vi "BRig_RT_comm_webdav_upload_all__announceExpPrefix.vi"(6 "input_fileName_prefix":string, 10 "input_errro":errorcluster, 11 "intput_hSession":T1) -> (0 "output_checkData":bool, 2 "output_error":errorcluster, 3 "output_hSession":T1)   [LabVIEW 2014]
uses:
  <vilib>/WebDAVClient/Advanced/SessionHandle.ctl
  <vilib>/WebDAVClient/NI_WebDAV.lvlib
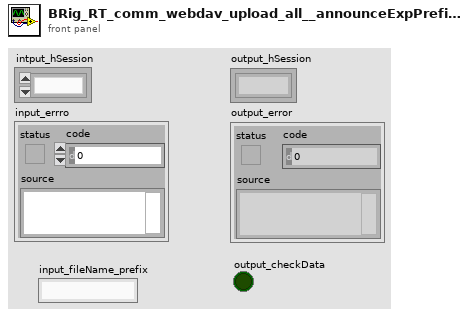
[diagram p1: front panel]
types:
  T1 = typedef "NI_WebDAV.lvlib/SessionHandle.ctl" = refnum<k1>
  T2 = enum16{"open", "replace", "create", "open or create", "replace or create", "replace or create with confirmation"}
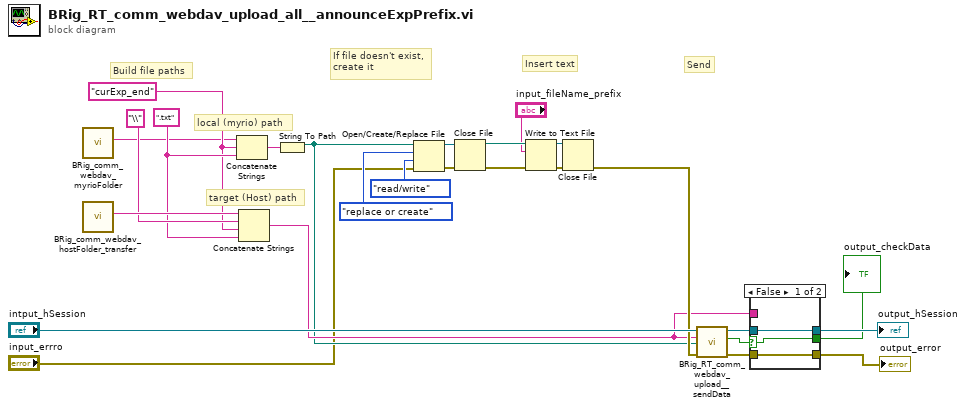
[diagram p0: block diagram]
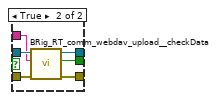
[diagram p2: hidden frame]
diagram:
  w22 = "curExp_end" ("intput_fileName")
  w23 = ".txt" ("string")
  # "Send"
  # "Insert text"
  # "If file doesn't exist,\ncreate it"
  # "local (myrio) path"
  # "target (Host) path"
  # "Build file paths"
  n1 = call "BRig_comm_webdav_myrioFolder.vi"() -> ("output_myrioFolder"=w21:string)  [unwired: 11 in]
  n2 = call "BRig_comm_webdav_hostFolder_transfer.vi"() -> ("output_HostFolder"=w25:string)  [unwired: 11 in]
  n3 = Concatenate Strings(w21, w22, w23) -> (w26:string)
  n4 = Concatenate Strings(w25, "\\" ("string"), w22, w23) -> (w10:string)
  n5 = String To Path(string=w26) -> (path=w2:path)
  n6 = Open/Create/Replace File(file path (use dialog)=w2, error in="input_errro", operation (0:open)=T2."replace or create", access (0:read/write)=enum16{"read/write", "read-only", "write-only"}."read/write") -> (refnum out=w3:refnum<file>, error out=w4:errorcluster)  [unwired: 2 in, 1 out]
  n7 = Close File(refnum=w3, error in=w4) -> (path=w17:path, error out=w18:errorcluster)
  n8 = Write to Text File(file (use dialog)=w17, text="input_fileName_prefix", error in=w18) -> (refnum out=w20:refnum<file>, error out=w19:errorcluster)  [unwired: 1 in, 1 out]
  n9 = Close File(refnum=w20, error in=w19) -> (error out=w14:errorcluster)  [unwired: 1 out]
  n10 = call "BRig_RT_comm_webdav_upload__sendData.vi"("input_error"=w14, "input_localPath"=w2, "input_targetPath"=w10, "input_hSession"="intput_hSession") -> ("error out"=w11:errorcluster, "output_sendData"=w12:bool, "output_hSession"=w13:T1)  [unwired: 5 in]
  n11 = case shown="False" w12 {
    selector: w12 -> [w27 _]
    tunnel: w13 -> [w29 w35]
    tunnel: w11 -> [w28 w34]
    tunnel: w10 -> [_ w33]
    tunnel: [w29 w32] -> w9
    tunnel: [w28 w31] -> w8
    tunnel: [w27 w30] -> w7
    frame False {
    }
    frame True {
      n12 = call "BRig_RT_comm_webdav_upload__checkData.vi"("input_error"=w34, "input_targetPath"=w33, "input_hSession"=w35) -> ("error out"=w31:errorcluster, "output_checkData"=w30:bool, "output_hSession"=w32:T1)  [unwired: 6 in]
    }
  }
  "output_hSession" <- w9
  "output_error" <- w8
  "output_checkData" <- w7
